vi "Leaktest Rescale Chart x v6.vi"(0 "Absolute Pres Cht Ref":refnum<vi>, 1 "Chart Hrs":dbl=0.5 min=0.25 max=24.0 step=0.25, 3 "Chart Zero":dbl=0.25 min=0.0 max=23.0 step=0.25, 5 "Diff Pres Cht Ref":refnum<vi>, 7 "Temp Cht Ref":refnum<vi>, 9 "Heat % Cht ref":refnum<vi>, 11 "error in (no error)":errorcluster, 12 "X Mult sec":u32) -> (15 "error out":errorcluster)   [LabVIEW 2020]
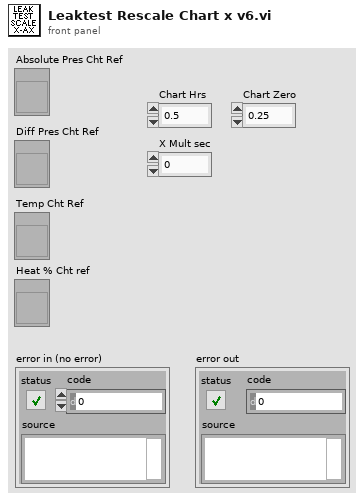
[diagram p1: front panel]
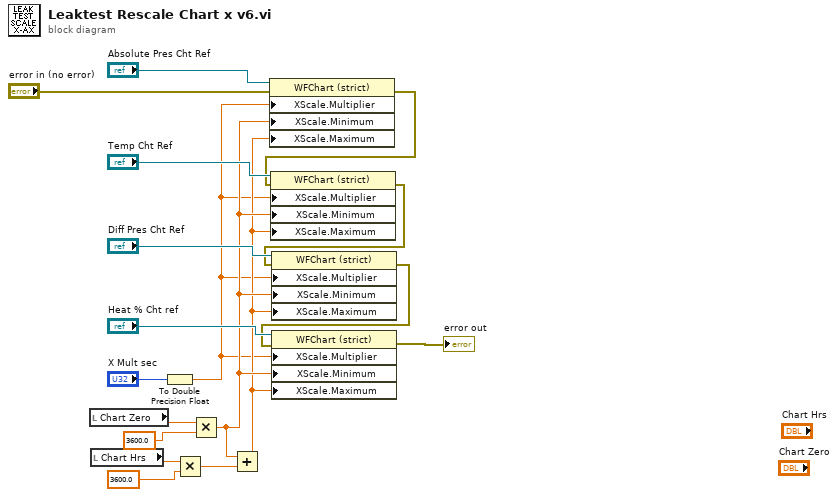
[diagram p0: block diagram]
diagram:
  n1 = local read "Chart Zero"() -> (w14:dbl)
  n2 = local read "Chart Hrs"() -> (w13:dbl)
  n3 = To Double Precision Float(number="X Mult sec") -> (double precision float=w1:dbl)
  n4 = Multiply(x=w13, y=3600.0) -> (x*y=w9:dbl)
  n5 = Multiply(x=w14, y=3600.0) -> (x*y=w10:dbl)
  n6 = Add(x=w10, y=w9) -> (x+y=w8:dbl)
  n7 = property class="WFChart (strict)"(reference="Absolute Pres Cht Ref", error in="error in (no error)", "XScale.Multiplier"=w1, "XScale.Minimum"=w10, "XScale.Maximum"=w8) -> (error out=w5:errorcluster)  [unwired: 1 out]
  n8 = property class="WFChart (strict)"(reference="Temp Cht Ref", error in=w5, "XScale.Multiplier"=w1, "XScale.Minimum"=w10, "XScale.Maximum"=w8) -> (error out=w4:errorcluster)  [unwired: 1 out]
  n9 = property class="WFChart (strict)"(reference="Diff Pres Cht Ref", error in=w4, "XScale.Multiplier"=w1, "XScale.Minimum"=w10, "XScale.Maximum"=w8) -> (error out=w3:errorcluster)  [unwired: 1 out]
  n10 = property class="WFChart (strict)"(reference="Heat % Cht ref", error in=w3, "XScale.Multiplier"=w1, "XScale.Minimum"=w10, "XScale.Maximum"=w8) -> (error out=→"error out":errorcluster)  [unwired: 1 out]
